vi "interlock_ctrl.vi"(7 "Interlock":bool) -> ()   [LabVIEW 2019]
uses:
  <vilib>/myRIO/Instrument Drivers/Onboard IO/UART/typedef/VISA Configuration.ctl
  <vilib>/Instr/_visa.llb/VISA Configure Serial Port (Instr).vi
  <vilib>/myRIO/Instrument Drivers/Onboard IO/UART/UART.lvlib
panel:
  out "resulting string":string
  out "Characters Read":string
  out "Character Count":u32
  in  "error in (no error)":errorcluster
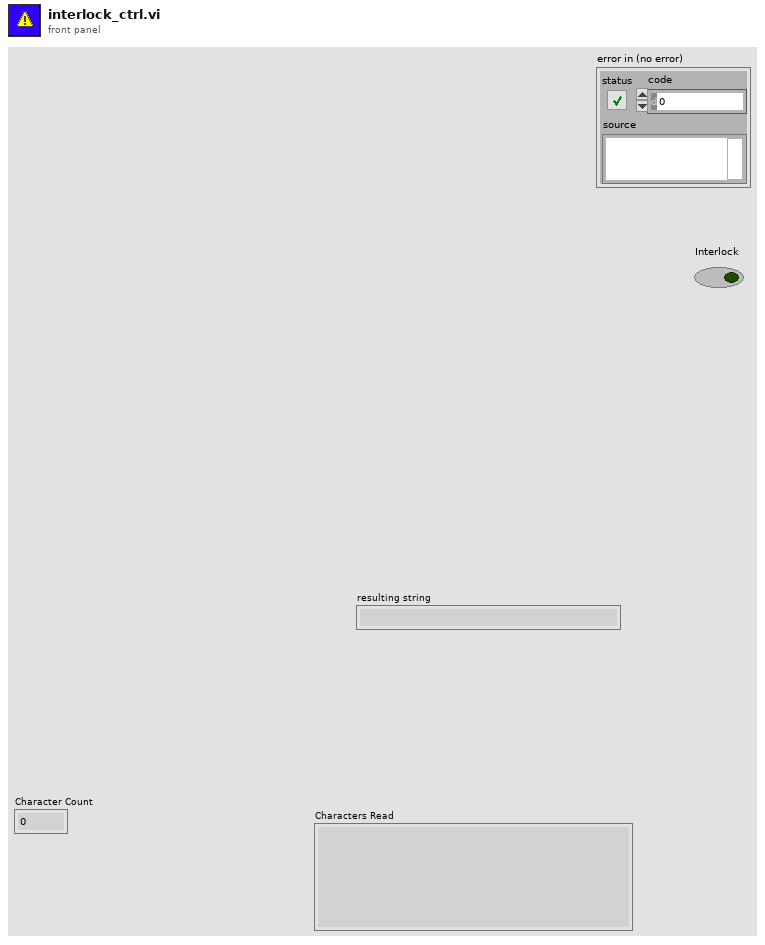
[diagram p1: front panel]
types:
  T1 = typedef "UART.lvlib/VISA Configuration.ctl" = cluster{"baud rate (9600)":u32, "data bits (8)":u16, "parity (0:none)":enum16{"None", "Odd", "Even", "Mark", "Space"}, "stop bits (10: 1 bit)":u16, "flow control (0:none)":u16, "termination char\n(0xA = '\\n' = LF) ":u8, "Enable Termination\nChar (T)":bool, "timeout (10sec)":u32}
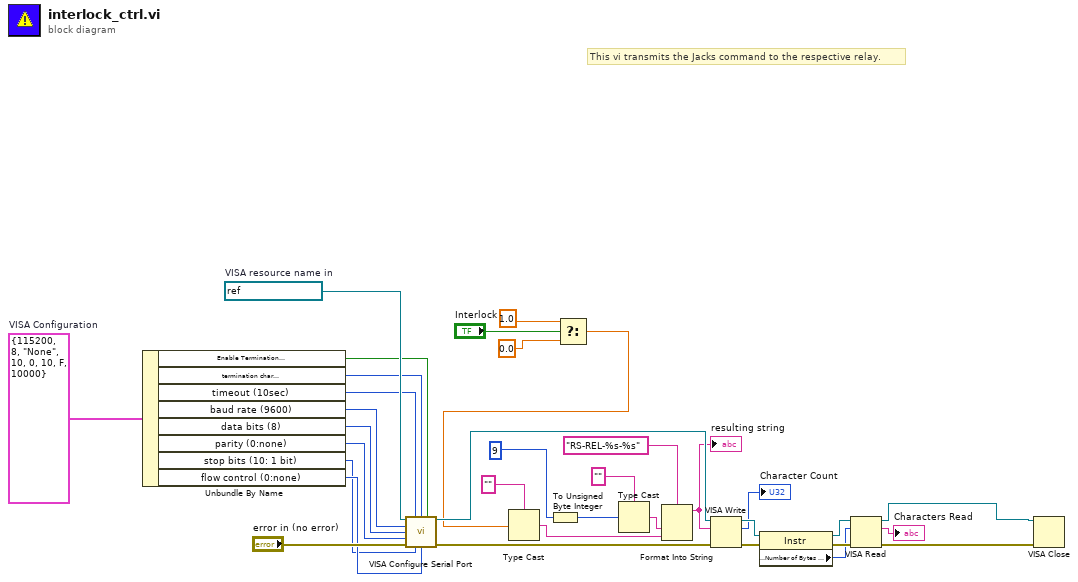
[diagram p0: block diagram]
diagram:
  w33 = T1 {"baud rate (9600)"=115200, "data bits (8)"=8, "parity (0:none)"=enum."None", "stop bits (10: 1 bit)"=10, "flow control (0:none)"=0, "termination char\n(0xA = '\\n' = LF) "=10, "Enable Termination\nChar (T)"=FALSE, "timeout (10sec)"=10000}  # VISA Configuration
  w34 = refnum<visa-resource-name> "ASRL2::INSTR"  # VISA resource name in
  # "This vi transmits the Jacks command to the respective relay."
  n1 = Unbundle By Name(w33) -> ("Enable Termination\nChar (T)"=w31:bool, "termination char\n(0xA = '\\n' = LF)"=w30:u8, "timeout (10sec)"=w29:u32, "baud rate (9600)"=w24:u32, "data bits (8)"=w25:u16, "parity (0:none)"=w26:enum16{"None", "Odd", "Even", "Mark", "Space"}, "stop bits (10: 1 bit)"=w27:u16, "flow control (0:none)"=w28:u16)
  n2 = call-poly "VISA Configure Serial Port"("VISA resource name"=w34, "timeout (10sec)"=w29, "termination char\n(0xA = '\\n' = LF)"=w30, "Enable Termination\nChar (T)"=w31, "baud rate (9600)"=w24, "data bits (8)"=w25, "parity (0:none)"=w26, "error in (no error)"="error in (no error)", "stop bits (10: 1 bit)"=w27, "flow control (0:none)"=w28) -> ("VISA resource name out"=w22:refnum<visa-resource-name>, "error out"=w18:errorcluster)  [unwired: 4 in]
  n3 = To Unsigned Byte Integer(number=u8 9) -> (unsigned 8bit integer=w17:u8)
  n4 = Select(t=1.0, s="Interlock", f=0.0) -> (s? t:f=w2:dbl)
  n5 = Type Cast(type="", x=w2) -> (*(type *) &x=w14:string)
  n6 = Type Cast(type="", x=w17) -> (*(type *) &x=w15:string)
  n7 = Format Into String(format string="RS-REL-%s-%s", w15, w14) -> (resulting string=w16:string)  [unwired: 2 in, 1 out]
  "resulting string" <- w16
  n8 = VISA Write(VISA resource name=w22, write buffer=w16, error in (no error)=w18) -> (VISA resource name out=w11:refnum<visa-resource-name>, return count=→"Character Count":u32, error out=w12:errorcluster)
  n9 = property class="Instr"(reference=w11, error in=w12) -> (reference out=w10:refnum<visa-resource-name>, error out=w13:errorcluster, "Serial Settings:Number of Bytes at Serial Port"=w9:u32)
  n10 = VISA Read(VISA resource name=w10, byte count=w9, error in (no error)=w13) -> (VISA resource name out=w20:refnum<visa-resource-name>, read buffer=→"Characters Read":string, error out=w19:errorcluster)  [unwired: 1 out]
  n11 = VISA Close(VISA resource name=w20, error in (no error)=w19) -> ()  [unwired: 1 out]
